vi "Move tail.vi"(9 "T":i32[](array[numeric])=[0, 0], 11 "H":i32[](array[numeric])=[0, 0]) -> (1 "T 2":i32[](array[numeric]))   [LabVIEW 2020]
uses:
  6f7abd9f-e08e-476d-a6d4-5831ec81c6e5.vi
  <vilib>/Comparison/Equal/Equal Functor/Equal Functor.lvclass
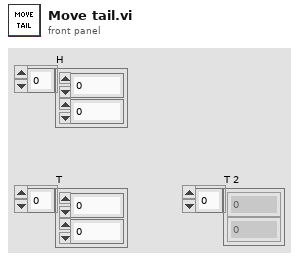
[diagram p1: front panel]
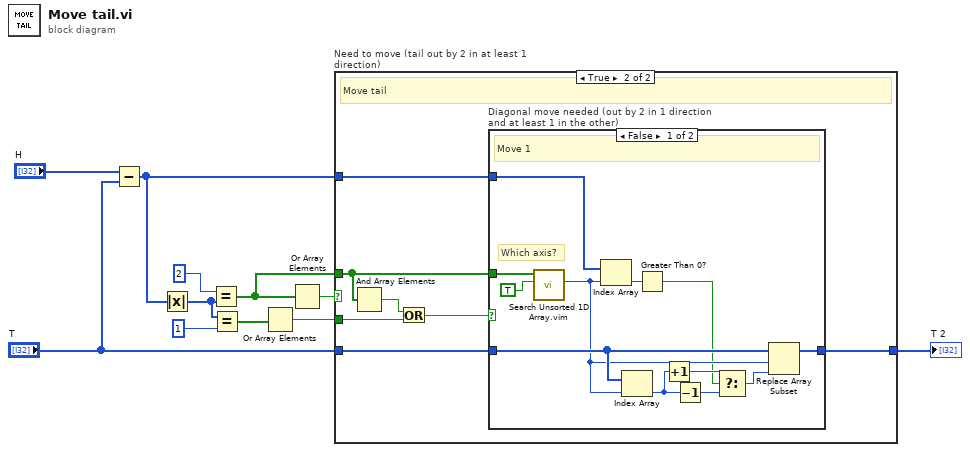
[diagram p0: block diagram]
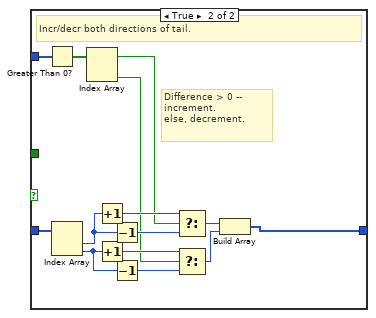
[diagram p3: hidden frame]
diagram:
  n1 = Subtract(x="H", y="T") -> (x-y=w8:i32[])
  n2 = Absolute Value(x=w8) -> (abs(x)=w5:i32[])
  n3 = Equal?(x=2, y=w5) -> (x = y?=w1:bool[])
  n4 = Equal?(x=w5, y=1) -> (x = y?=w3:bool[])
  n5 = Or Array Elements(Boolean array=w3) -> (logical OR=w2:bool)
  n6 = Or Array Elements(Boolean array=w1) -> (logical OR=w6:bool)
  n7 = case "Need to move (tail out by 2 in at least 1 direction)" shown="True" w6 {
    tunnel: [w12 w16] -> w9
    tunnel: "T" -> [w12 w18]
    tunnel: w8 -> [_ w19]
    tunnel: w2 -> [_ w17]
    tunnel: w1 -> [_ w14]
    frame False {
    }
    frame True {
      # "Move tail"
      n8 = And Array Elements(Boolean array=w14) -> (logical AND=w13:bool)
      n9 = Or(x=w13, y=w17) -> (x .or. y?=w15:bool)
      n10 = case "Diagonal move needed (out by 2 in 1 direction and at least 1 in the other)" shown="False" w15 {
        tunnel: w19 -> [w29 w35]
        tunnel: w18 -> [w28 w45]
        tunnel: [w26 w37] -> w16
        tunnel: w14 -> [w31 _]
        frame False {
          # "Which axis?"
          # "Move 1"
          n11 = call "Search Unsorted 1D Array.vim"("element"=TRUE, "unsorted 1D array"=w31) -> ("index of element"=w27:i32)  [unwired: 9 in]
          n12 = Index Array(array=w29, index=w27) -> (element=w21:i32)
          n13 = Index Array(array=w28, index=w27) -> (element=w23:i32)
          n14 = Greater Than 0?(x=w21) -> (x > 0?=w20:bool)
          n15 = Increment(x=w23) -> (x+1=w25:i32)
          n16 = Decrement(x=w23) -> (x-1=w24:i32)
          n17 = Select(t=w25, s=w20, f=w24) -> (s? t:f=w22:i32)
          n18 = Replace Array Subset(array=w28, new element=w22, index=w27) -> (w26:i32[])
        }
        frame True {
          # "Difference > 0 -- increment.\nelse, decrement."
          # "Incr/decr both directions of tail."
          n19 = Greater Than 0?(x=w35) -> (x > 0?=w36:bool[])
          n20 = Index Array(array=w45) -> (element #1=w42:i32, element #2=w41:i32)  [unwired: 2 in]
          n21 = Index Array(array=w36) -> (element #1=w34:bool, element #2=w33:bool)  [unwired: 2 in]
          n22 = Increment(x=w42) -> (x+1=w44:i32)
          n23 = Increment(x=w41) -> (x+1=w40:i32)
          n24 = Decrement(x=w42) -> (x-1=w43:i32)
          n25 = Decrement(x=w41) -> (x-1=w39:i32)
          n26 = Select(t=w44, s=w34, f=w43) -> (s? t:f=w38:i32)
          n27 = Select(t=w40, s=w33, f=w39) -> (s? t:f=w32:i32)
          n28 = Build Array(w38, w32) -> (w37:i32[])
        }
      }
    }
  }
  "T 2" <- w9
